vi "LaserSetVotage.vi"(7 "error in (no error)":errorcluster, 10 "Config In":T1) -> (0 "error out":errorcluster, 2 "TIRFLock":cluster{"Time":dbl, "Votage":dbl}, 3 "Config Out":T1)   [LabVIEW 2019]
doc: "Generates sample waveforms according to the signal type in the HW Config input."
uses:
  Settings/Settings.ctl
  Support/Hardware Configuration.ctl
  Support/Camera Configuration.ctl
  E:/DevHardSoftware/MMicroscopy/HardwareAdapter/Camera/Dependencies/PVCamNET.dll
  Camera/Dependencies/PVCamNET.dll
  <vilib>/userdefined/High Color/IMAQdx.ctl
  E:/DevHardSoftware/MMicroscopy/HardwareAdapter/Lasers/Dependencies/Oxxius_Boxx.dll
  Dependencies/Oxxius_Boxx.dll
  Logging/Logging Configuration.ctl
  controls/UI Configuration.ctl
  <vilib>/numeric/Random Number (Range) U64.vi
  <vilib>/numeric/sub_Random U32.vi
  Logging/Logging.lvlib
  Settings/Settings.lvlib
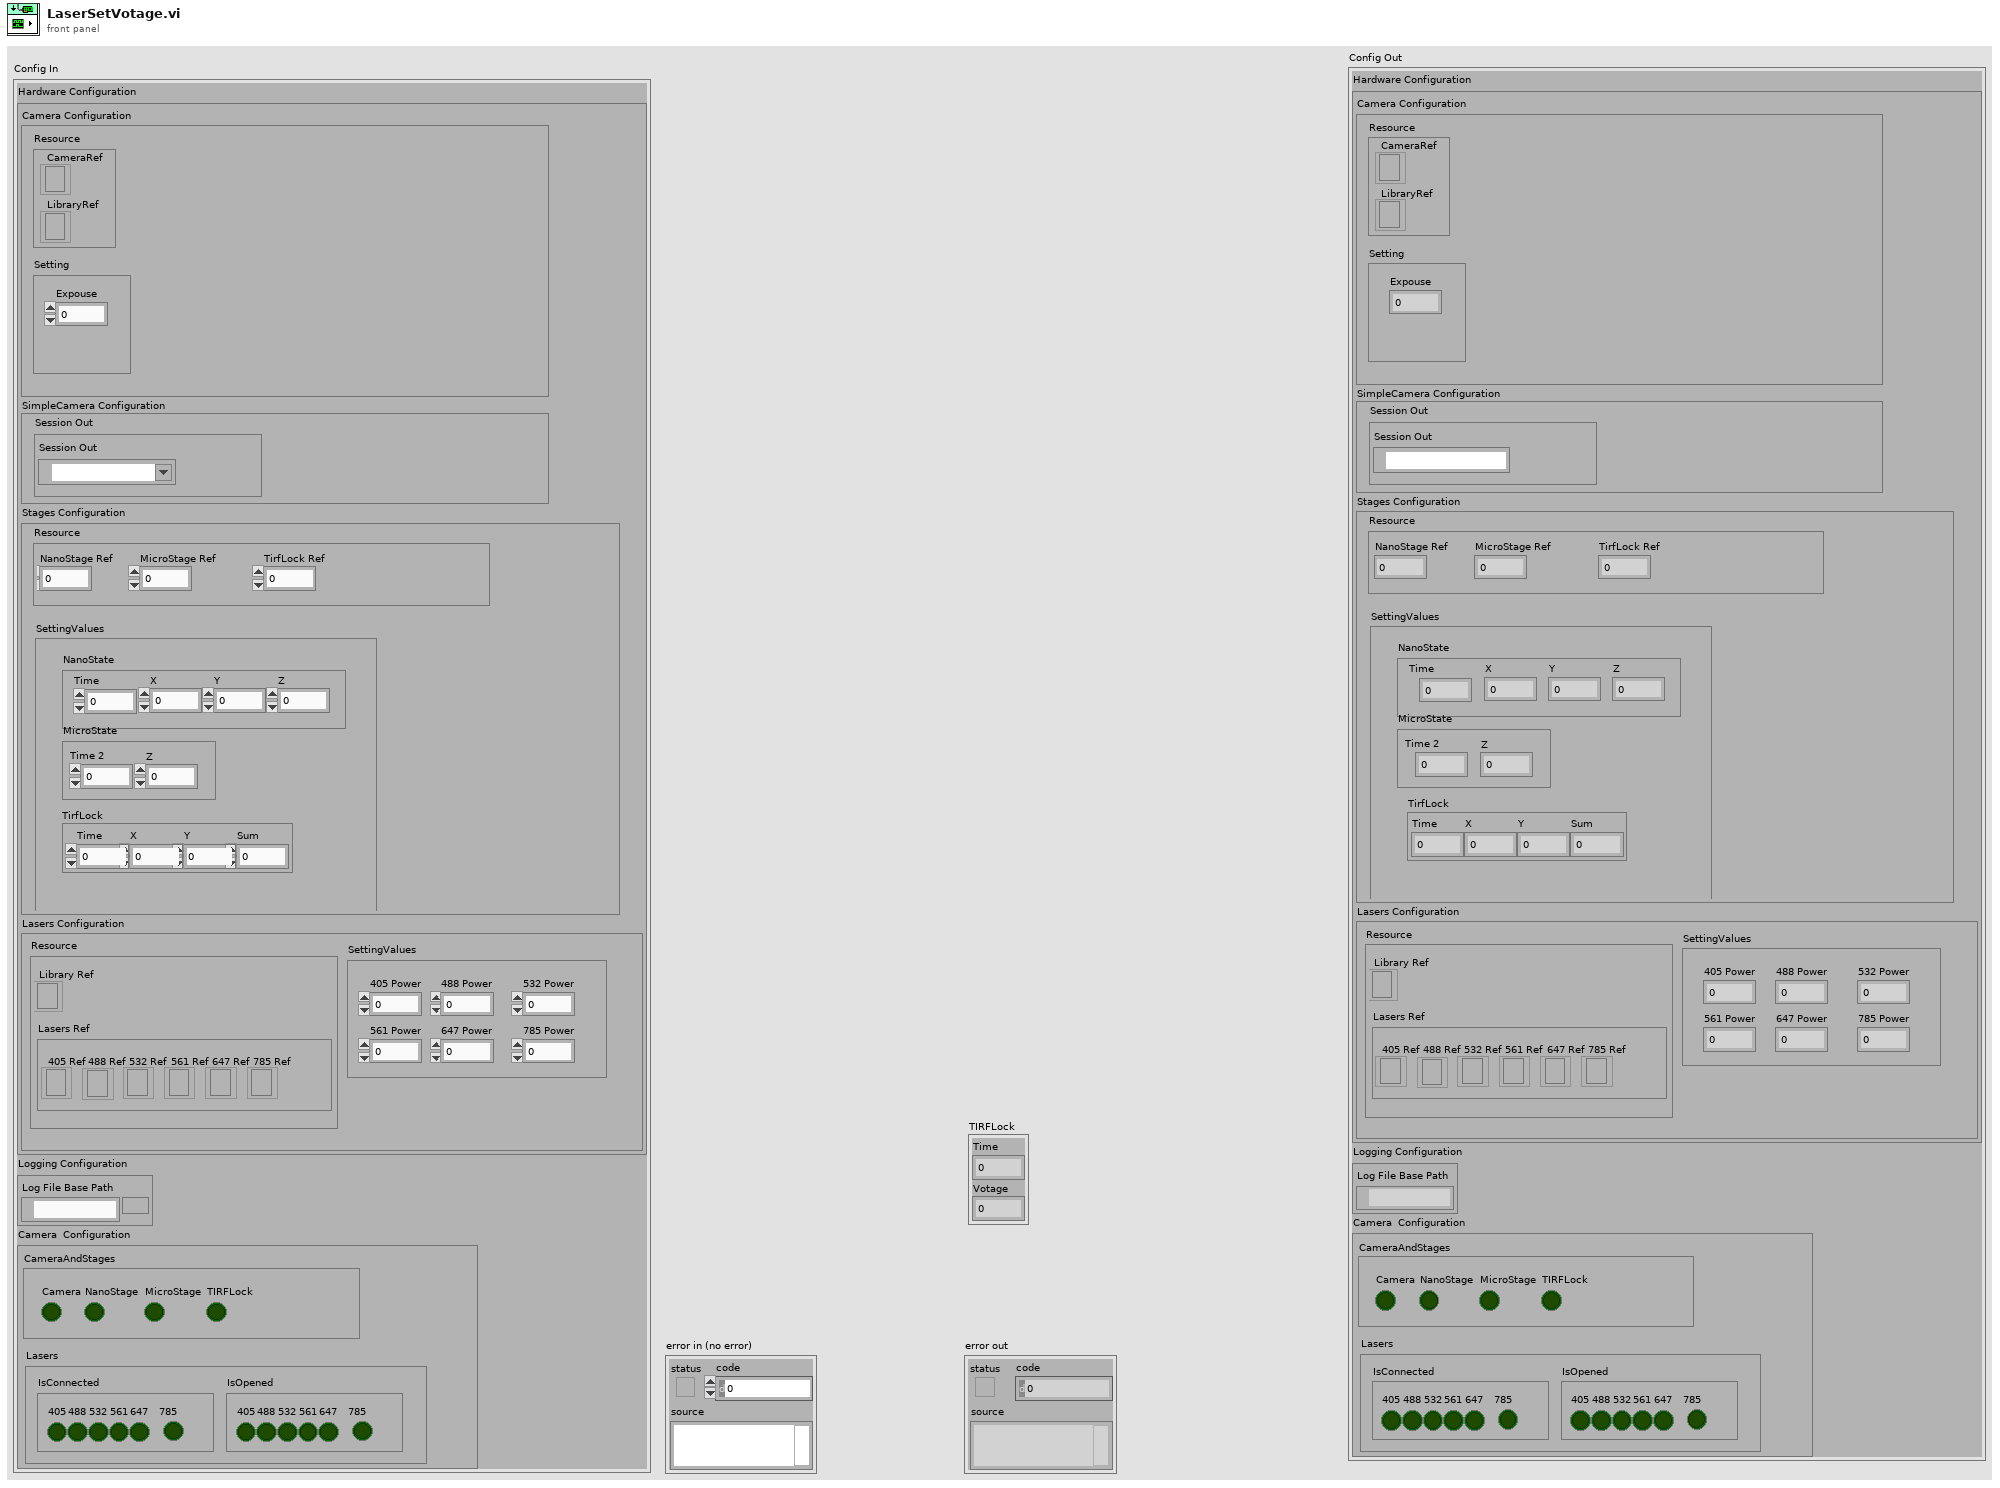
[diagram p1: front panel]
types:
  T1 = typedef "Settings.lvlib/Settings.ctl" = cluster{"Hardware Configuration":T2, "Logging Configuration":T5, "HardWare Status":cluster{"CameraAndStages":T6, "Lasers":cluster{"IsConnected":cluster{"405":bool, "488":bool, "532":bool, "561":bool, "647":bool, "785":bool}, "IsOpened":cluster{"405":bool, "488":bool, "532":bool, "561":bool, "647":bool, "785":bool}}}}
  T2 = typedef "Hardware Configuration.ctl" = cluster{"Camera Configuration":T3, "SimpleCamera Configuration":cluster{"Resource":cluster{"Session Out":T4}}, "Stages Configuration":cluster{"Resource":cluster{"NanoStage Ref":i32, "MicroStage Ref":i32, "TirfLock Ref":i32}, "SettingValues":cluster{"NanoState":cluster{"Time":dbl, "X":dbl, "Y":dbl, "Z":dbl}, "MicroState":cluster{"Time 2":dbl, "Z":dbl}, "TirfLock":cluster{"Time":dbl, "X":dbl, "Y":dbl, "Sum":dbl}}}, "Lasers Configuration":cluster{"SettingValues":cluster{"405 Power":i32, "488 Power":i32, "532 Power":i32, "561 Power":i32, "647 Power":i32, "785 Power":i32}, "Resource":cluster{"Library Ref":refnum<k24>, "Lasers Ref":cluster{"405 Ref":refnum<k24>, "488 Ref":refnum<k24>, "532 Ref":refnum<k24>, "561 Ref":refnum<k24>, "647 Ref":refnum<k24>, "785 Ref":refnum<k24>}}}}
  T3 = typedef "Camera Configuration.ctl" = cluster{"Resource":cluster{"CameraRef":refnum<k24>, "LibraryRef":refnum<k24>}, "Setting":cluster{"Expouse":dbl}}
  T4 = typedef "IMAQdx.ctl" = refnum<k21>
  T5 = typedef "Logging.lvlib/Logging Configuration.ctl" = cluster{"Log File Base Path":path}
  T6 = typedef "UI Configuration.ctl" = cluster{"Camera":bool, "NanoStage":bool, "MicroStage":bool, "TIRFLock":bool}
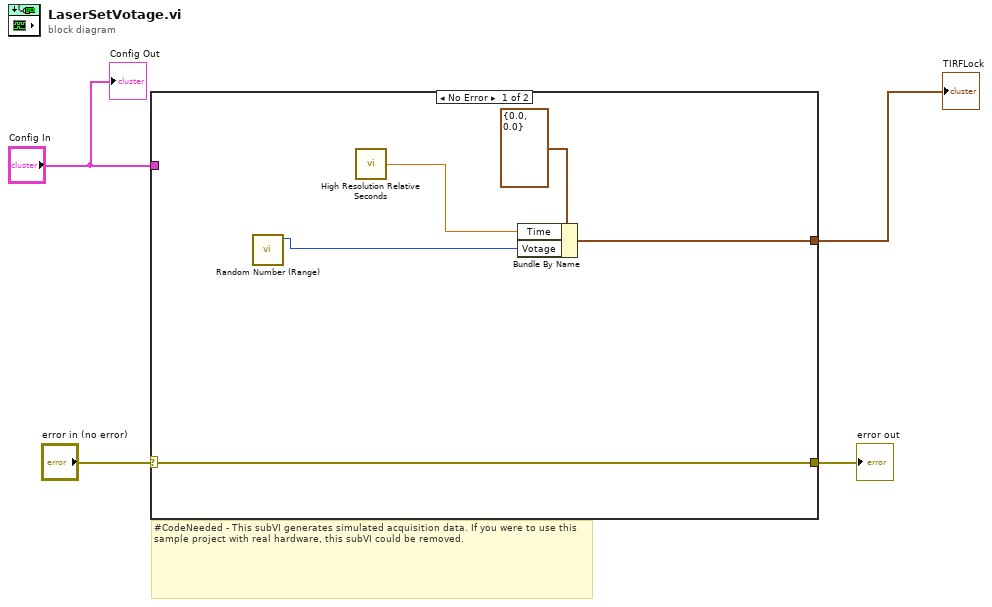
[diagram p0: block diagram]
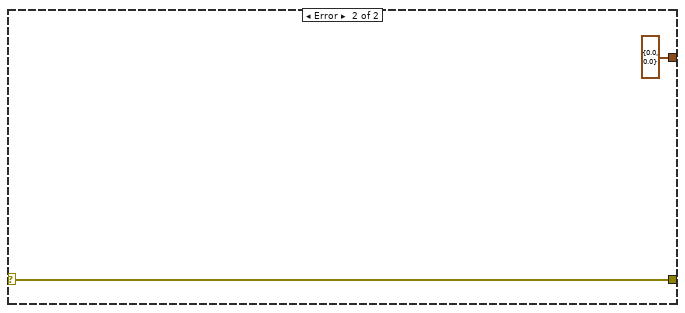
[diagram p2: hidden frame]
diagram:
  # "#CodeNeeded - This subVI generates simulated acquisition data. If you were to use this sample project with real hardware, this subVI could be removed."
  n1 = case shown="No Error" "error in (no error)" {
    selector: "error in (no error)" -> [w9 w11]
    tunnel: [w9 w11] -> w3
    tunnel: "Config In" -> [_ _]
    tunnel: [w5 cluster{"Time":dbl, "Votage":dbl} {"Time"=0.0, "Votage"=0.0} ("RawImage")] -> w1
    frame No Error {
      n2 = call-poly <vilib>:"Random Number (Range).vi"() -> ("number"=w6:u64)  [unwired: 11 in]
      n3 = call <vilib>:"High Resolution Relative Seconds.vi"() -> ("relative seconds"=w7:dbl)
      n4 = Bundle By Name(cluster=cluster{"Time":dbl, "Votage":dbl} {"Time"=0.0, "Votage"=0.0} ("RawImage"), "Time"=w7, "Votage"=w6) -> (w5:cluster{"Time":dbl, "Votage":dbl})
    }
    frame Error {
    }
  }
  "error out" <- w3
  "TIRFLock" <- w1
  "Config Out" <- "Config In"
